vi "Initialize Array from Array Example 01.vi"() -> ()   [LabVIEW 2009]
uses:
  Initialize Array from Array/Initialize 1D Array (Boolean) from 1D Array (String).vi
panel:
  in  "stop":bool
  in  "Array":bool[](array[boolean])
  in  "Names":string[](array[string])=["Frank", "Alice", "Raphael", "Walter", "Beatrice", "Harry", "Diane", "Cleo", "Lester"]
  # "Add or remove names here"
  # "Watch what happens here"
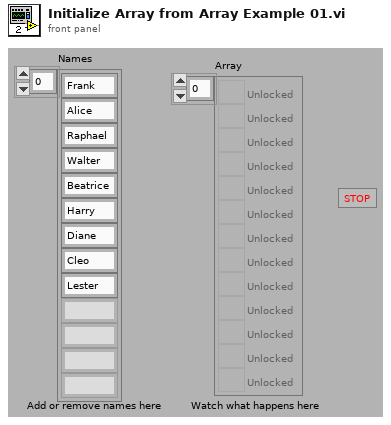
[diagram p1: front panel]
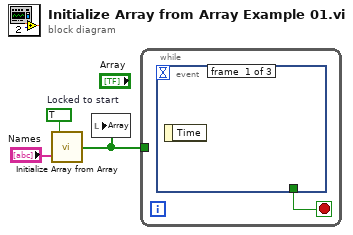
[diagram p0: block diagram]
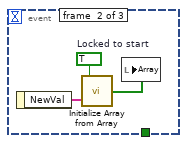
[diagram p2: hidden frame]
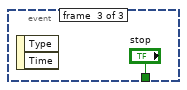
[diagram p3: hidden frame]
diagram:
  w2 = TRUE  # Locked to start
  n1 = call-poly "Initialize Array from Array.vi"("Input Array"="Names", "Element Data"=w2) -> ("Output Array"=w1:bool[])
  n2 = local write "Array"(w1) -> ()
  n3 = while {
    tunnel: w1 -> [_]
    stop <- w4 stop-if-true
    n4 = event shown="[1] \"Names\": Value Change" {
      selector: _ -> [_ _ _]
      dyn-events: _ -> [_ _ _]
      timeout: _ -> [_ _ _]
      tunnel: [_ _ "stop"] -> w4
      event #0 {
        n5 = event-data() -> ()  [unwired: 1 in, 1 out]
      }
      event #1 {
        w6 = TRUE  # Locked to start
        n6 = event-data() -> ("NewVal"=w5:string[])  [unwired: 1 in]
        n7 = call-poly "Initialize Array from Array.vi"("Input Array"=w5, "Element Data"=w6) -> ("Output Array"=w7:bool[])
        n8 = local write "Array"(w7) -> ()
      }
      event #2 {
        n9 = event-data() -> ()  [unwired: 1 in, 2 out]
      }
    }
  }
